vi "DecodeSignalSpecLine.vi"(8 "error in (no error)":errorcluster, 11 "Signal Spec Line":string) -> (0 "error out":errorcluster, 3 "Signal Spec Info":T1)   [LabVIEW 2012]
doc: "Decodes information about specified signal in .hea file."
uses:
  #TD_SignalSpecInfo.ctl
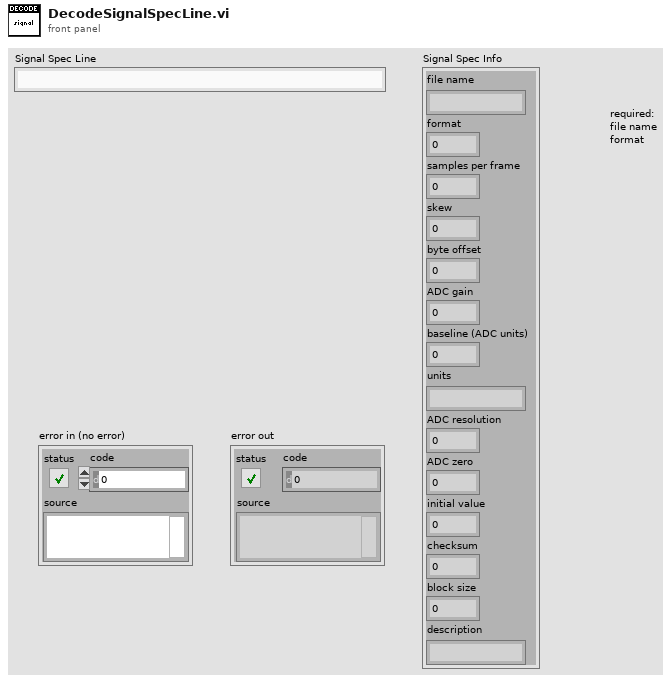
[diagram p1: front panel]
types:
  T1 = typedef "#TD_SignalSpecInfo.ctl" = cluster{"file name":string, "format":i32, "samples per frame":i32, "skew":i32, "byte offset":i32, "ADC gain":dbl, "baseline (ADC units)":i16, "units":string, "ADC resolution":i16, "ADC zero":i16, "initial value":i16, "checksum":i16, "block size":i32, "description":string}
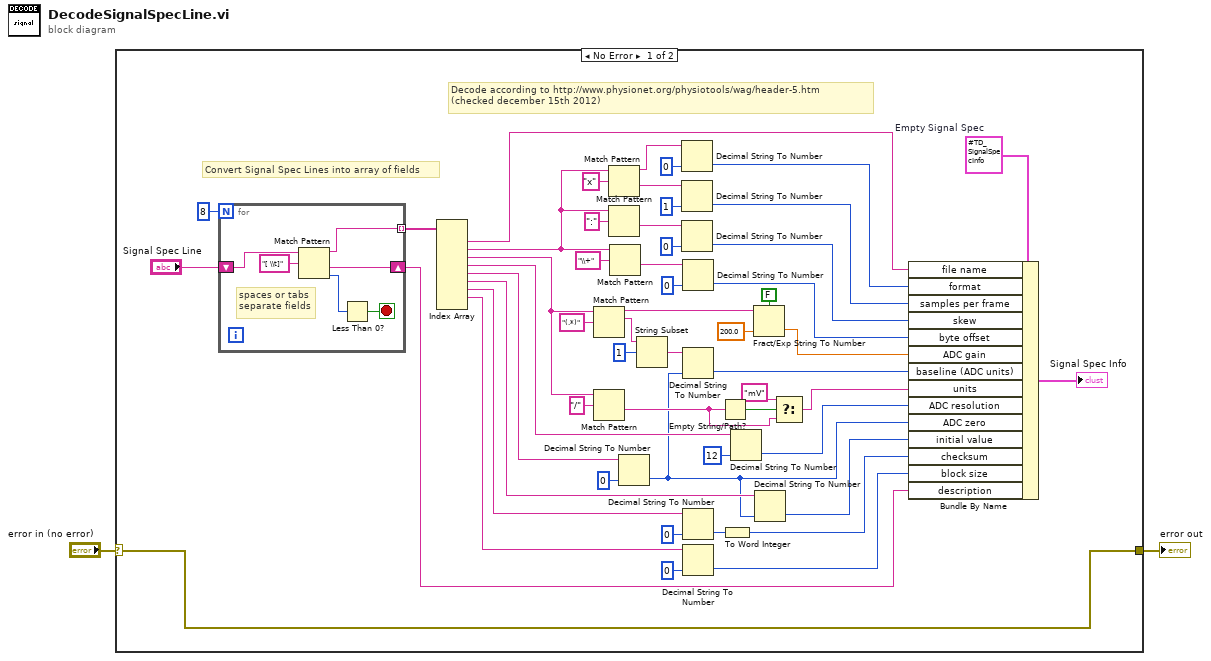
[diagram p0: block diagram]
diagram:
  n1 = case shown="No Error" "error in (no error)" {
    selector: "error in (no error)" -> [w13 w63]
    tunnel: [w13 w63] -> w1
    frame No Error {
      w56 = T1 {"file name"="", "format"=0, "samples per frame"=0, "skew"=0, "byte offset"=0, "ADC gain"=0.0, "baseline (ADC units)"=0, "units"="", "ADC resolution"=0, "ADC zero"=0, "initial value"=0, "checksum"=0, "block size"=0, "description"=""}  # Empty Signal Spec
      # "Decode according to http://www.physionet.org/physiotools/wag/header-5.htm\n(checked december 15th 2012)"
      # "Convert Signal Spec Lines into array of fields"
      n2 = for {
        N: 8 -> [_]
        shift-right: [w59] -> w10
        shift-left: "Signal Spec Line" -> [w62]
        tunnel: [w58] -> w12 mode=indexing
        stop <- w57 stop-if-true
        # "spaces or tabs\nseparate fields"
        n3 = Match Pattern(string=w62, regular expression="[ \\t]") -> (before substring=w58:string, after substring=w59:string, offset past match=w61:i32)  [unwired: 1 in, 1 out]
        n4 = Less Than 0?(x=w61) -> (x < 0?=w57:bool)
      }
      n5 = Index Array(array=w12) -> (element #1=w35:string, element #2=w41:string, element #3=w32:string, element #4=w26:string, element #5=w24:string, element #6=w22:string, element #7=w20:string, element #8=w16:string)  [unwired: 9 in, 1 out]
      n6 = Match Pattern(string=w32, regular expression="(.*)") -> (before substring=w37:string, match substring=w7:string)  [unwired: 1 in, 2 out]
      n7 = Match Pattern(string=w32, regular expression="/") -> (after substring=w30:string)  [unwired: 1 in, 3 out]
      n8 = Match Pattern(string=w41, regular expression="x") -> (before substring=w53:string, after substring=w50:string)  [unwired: 1 in, 2 out]
      n9 = Match Pattern(string=w41, regular expression=":") -> (after substring=w48:string)  [unwired: 1 in, 3 out]
      n10 = Match Pattern(string=w41, regular expression="\\+") -> (after substring=w42:string)  [unwired: 1 in, 3 out]
      n11 = Decimal String To Number(string=w24, default (0L)=i16 0 ("default (0 I32)")) -> (number=w9:i16)  [unwired: 1 in, 1 out]
      n12 = String Subset(string=w7, offset (0)=1) -> (substring=w6:string)  [unwired: 1 in]
      n13 = Decimal String To Number(string=w53, default (0L)=0 ("default (0 I32)")) -> (number=w54:i32)  [unwired: 1 in, 1 out]
      n14 = Decimal String To Number(string=w50, default (0L)=1 ("default (0 I32)")) -> (number=w49:i32)  [unwired: 1 in, 1 out]
      n15 = Decimal String To Number(string=w48, default (0L)=0 ("default (0 I32)")) -> (number=w45:i32)  [unwired: 1 in, 1 out]
      n16 = Decimal String To Number(string=w42, default (0L)=0 ("default (0 I32)")) -> (number=w40:i32)  [unwired: 1 in, 1 out]
      n17 = Decimal String To Number(string=w6, default (0L)=w9) -> (number=w36:i16)  [unwired: 1 in, 1 out]
      n18 = Decimal String To Number(string=w20, default (0L)=0 ("default (0 I32)")) -> (number=w4:i32)  [unwired: 1 in, 1 out]
      n19 = Decimal String To Number(string=w16, default (0L)=0 ("default (0 I32)")) -> (number=w17:i32)  [unwired: 1 in, 1 out]
      n20 = Empty String/Path?(string/path=w30) -> (empty?=w31:bool)
      n21 = To Word Integer(number=w4) -> (16bit integer=w3:i16)
      n22 = Decimal String To Number(string=w26, default (0L)=i16 12 ("default (0 I32)")) -> (number=w25:i16)  [unwired: 1 in, 1 out]
      n23 = Fract/Exp String To Number(use system decimal point (T)=FALSE, string=w37, default (0 dbl)=200.0 ("default (0 DBL)")) -> (number=w38:dbl)  [unwired: 1 in, 1 out]
      n24 = Decimal String To Number(string=w22, default (0L)=w9) -> (number=w21:i16)  [unwired: 1 in, 1 out]
      n25 = Select(t="mV", s=w31, f=w30) -> (s? t:f=w29:string)
      n26 = Bundle By Name(cluster=w56, "file name"=w35, "format"=w54, "samples per frame"=w49, "skew"=w45, "byte offset"=w40, "ADC gain"=w38, "baseline (ADC units)"=w36, "units"=w29, "ADC resolution"=w25, "ADC zero"=w9, "initial value"=w21, "checksum"=w3, "block size"=w17, "description"=w10) -> (→"Signal Spec Info":T1)
    }
    frame Error {
    }
  }
  "error out" <- w1
